vi "SignUpView.vi"(1 "Exit Button":bool) -> (0 "error out":errorcluster caption="에러 출력")   [LabVIEW 2019]
uses:
  <vilib>/Utility/miscctls.llb/LVPointTypeDef.ctl
  03_Home/controller/pannelState.ctl
panel:
  in  "signUp":bool
  out "idChecK?":bool
  in  "정지":bool
  in  "cancelBtn":bool
  in  "signUpBtn":bool
  in  "idCheck":bool
  in  "loginIdForm":string
  in  "securityAnswerForm":string
  in  "userEmailForm":string
  in  "userPhoneForm":string
  in  "userNmForm":string
  in  "passwordCheckForm":string
  in  "passwordForm":string
  in  "securityQuestionForm":string(combo)
  in  "error in (no error)":errorcluster caption="에러 입력(에러 없음)"
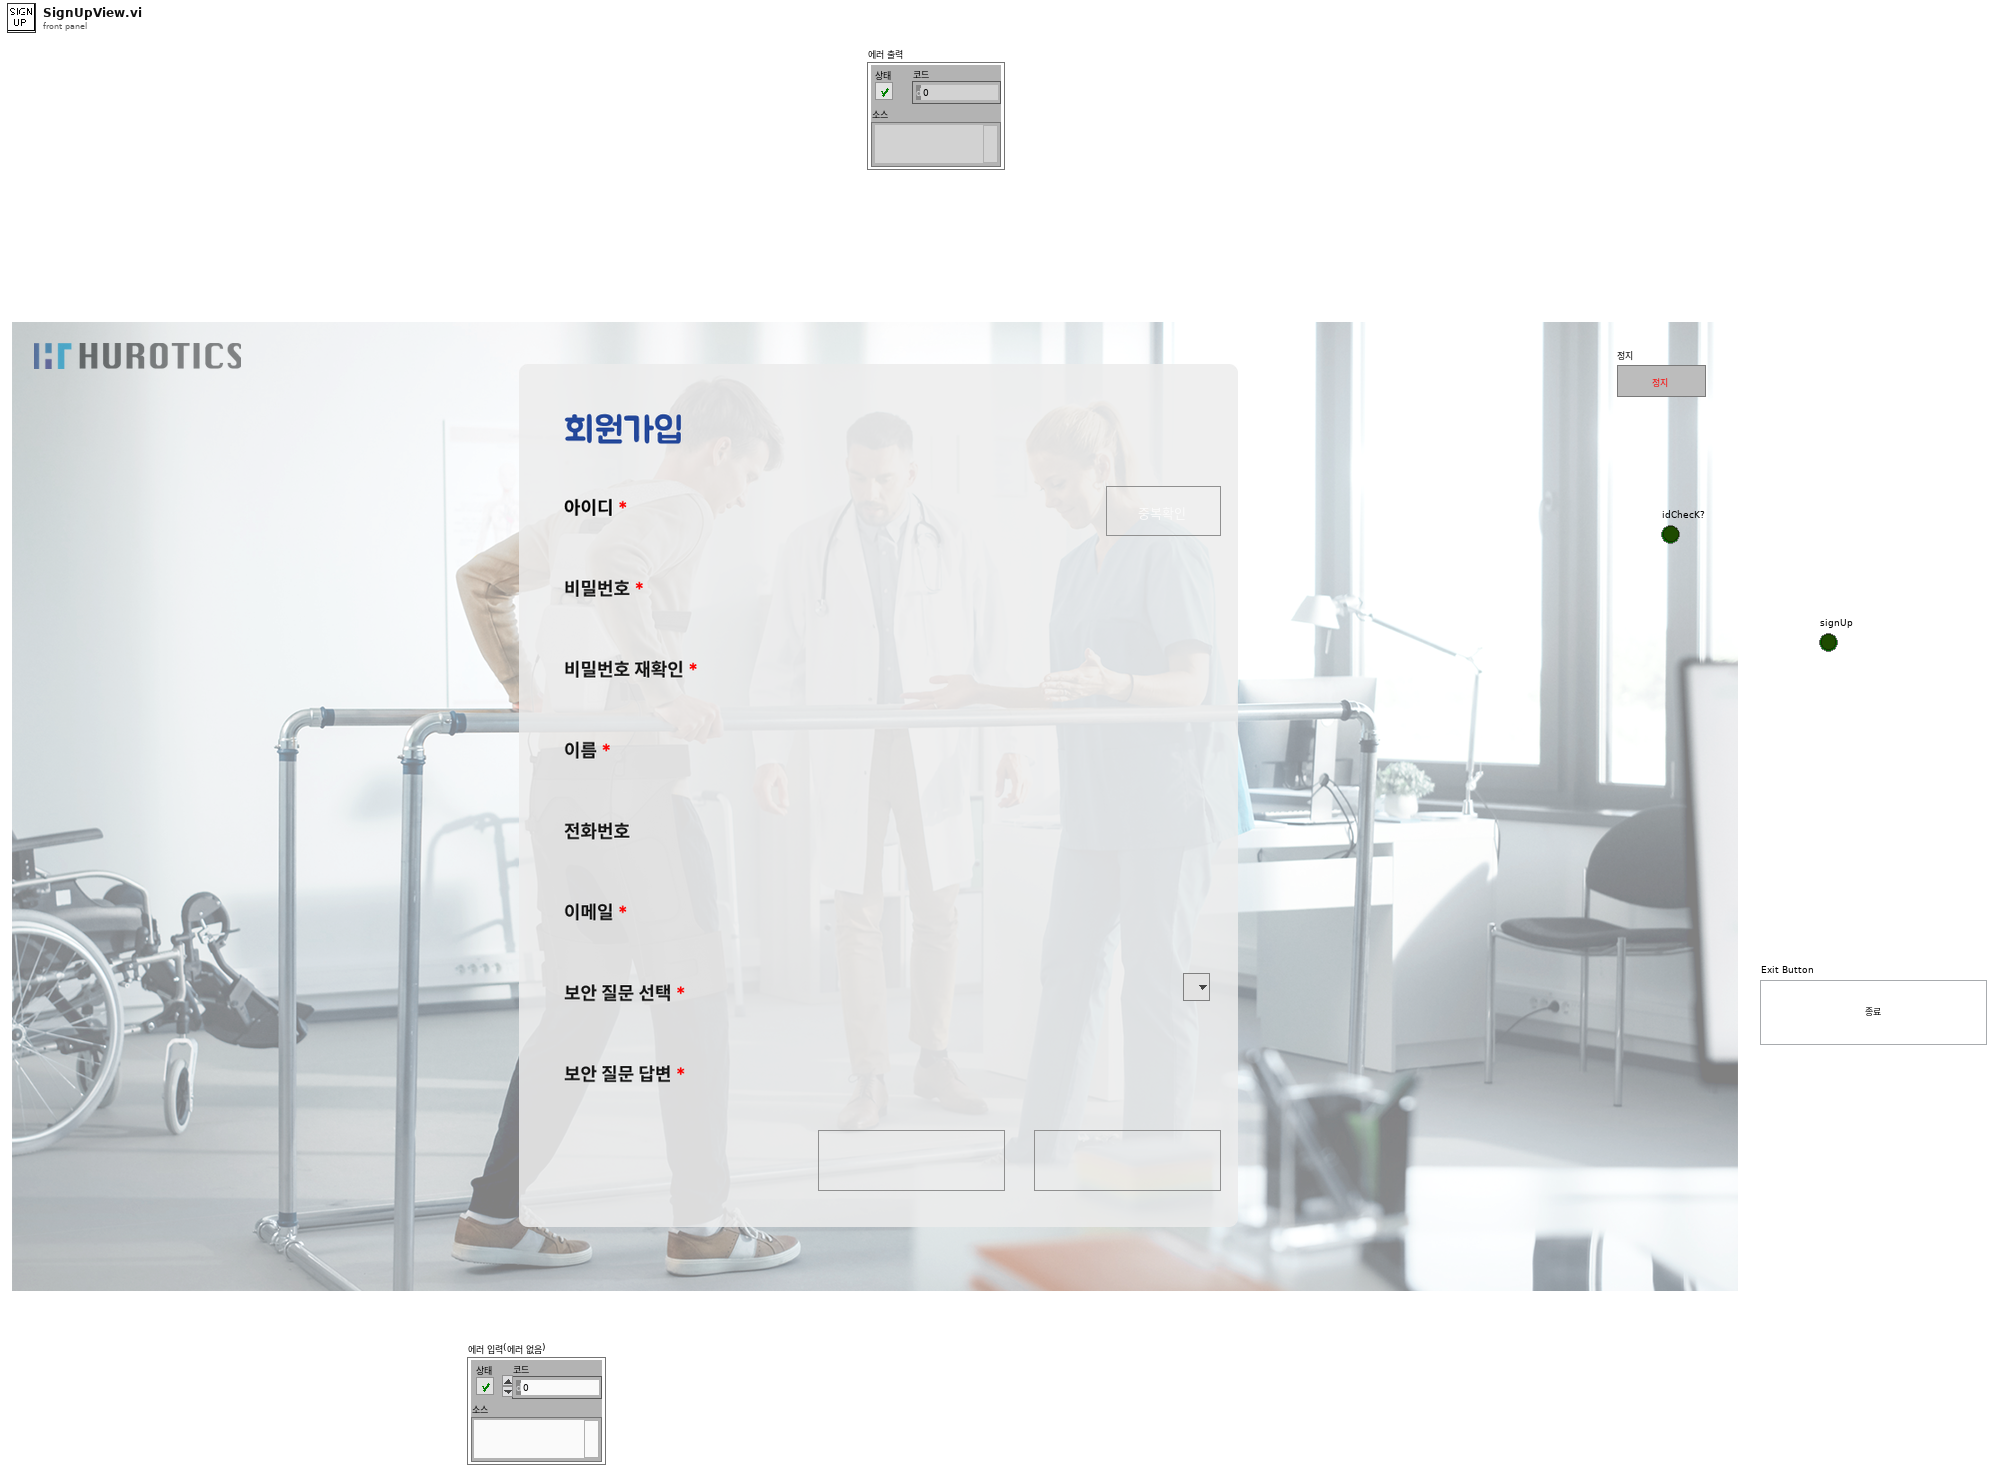
[diagram p1: front panel]
types:
  T1 = typedef "LVPointTypeDef.ctl" = cluster{"Horizontal":i16, "Vertical":i16}
  T2 = typedef "pannelState.ctl" = enum16{"Init", "LogIn", "SignUpView", "Home", "Management_patientList", "Management_patientTrashtList", "Management_patientCreate", "Management_patientUpdate", "Management_patientTraining", "Management_patientTrainingDetail", "H-MEDI PatientList", "H-MEDI HardwareCtl", "Adjust", "FineTuning", "UserList", "UserDetail", "Exit"}
  T3 = enum16{"connection", "create", "read", "update", "delete", "close"}
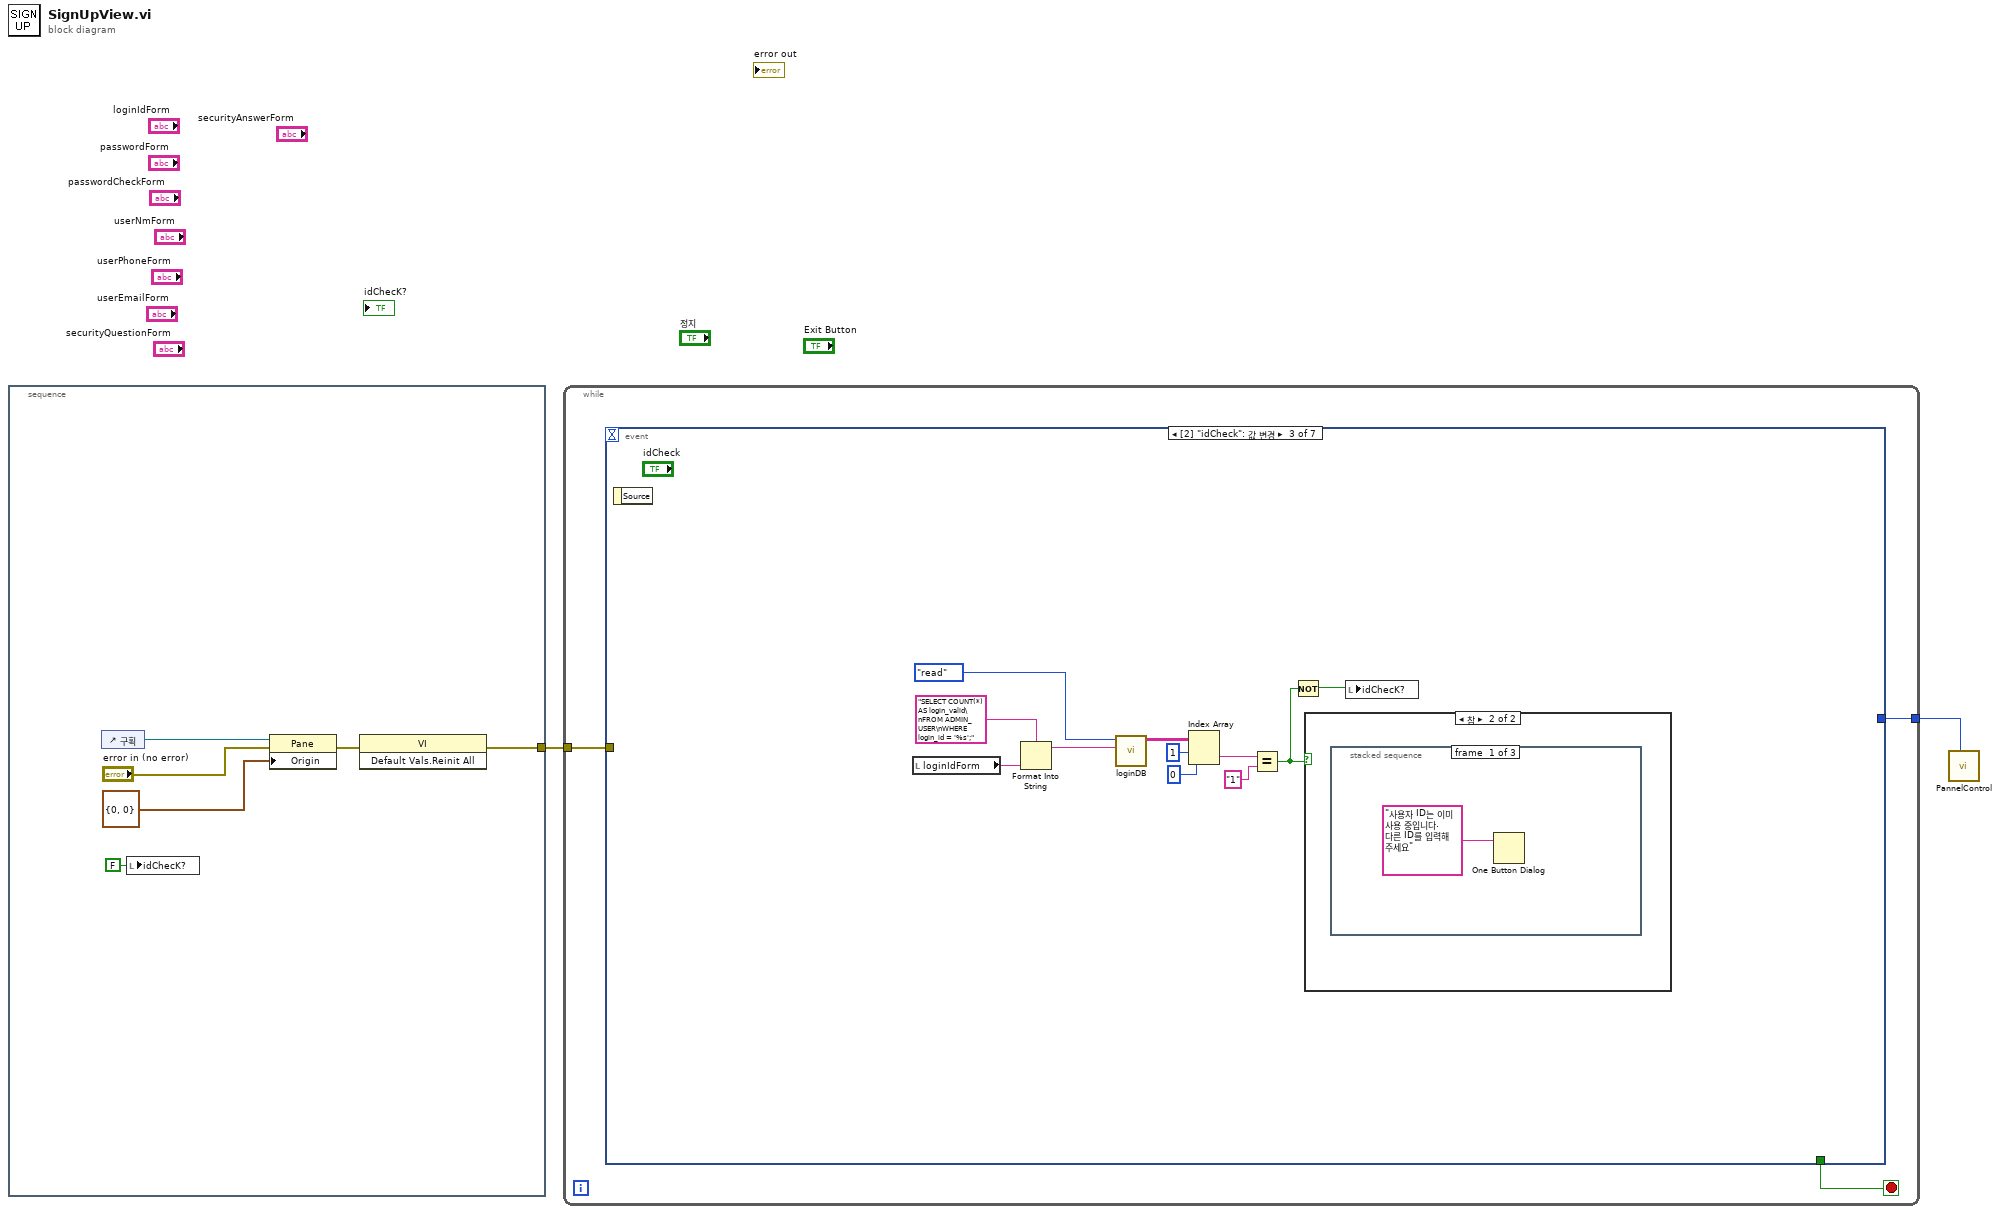
[diagram p0: block diagram]
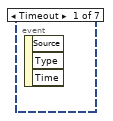
[diagram p2: hidden frame]
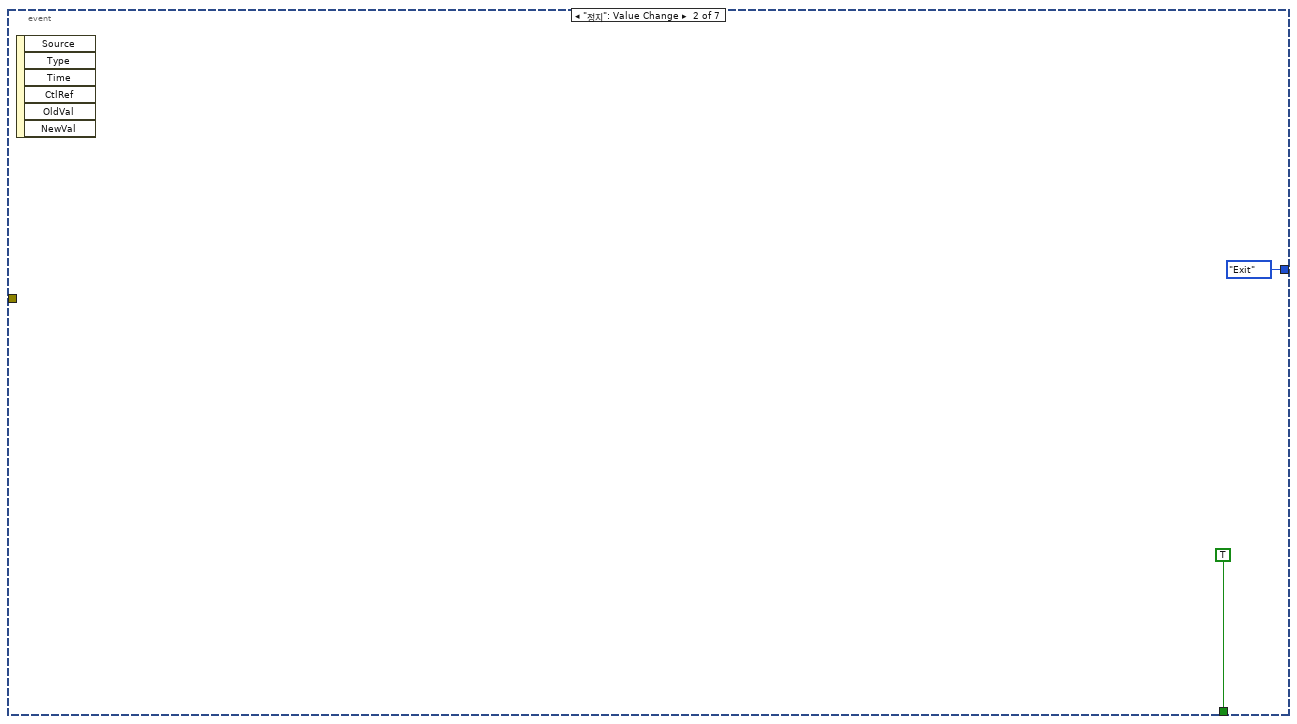
[diagram p3: hidden frame]
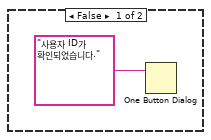
[diagram p4: hidden frame]
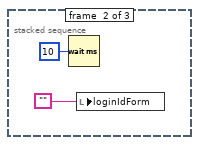
[diagram p5: hidden frame]
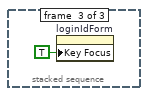
[diagram p6: hidden frame]
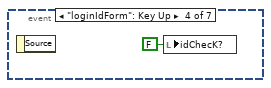
[diagram p7: hidden frame]
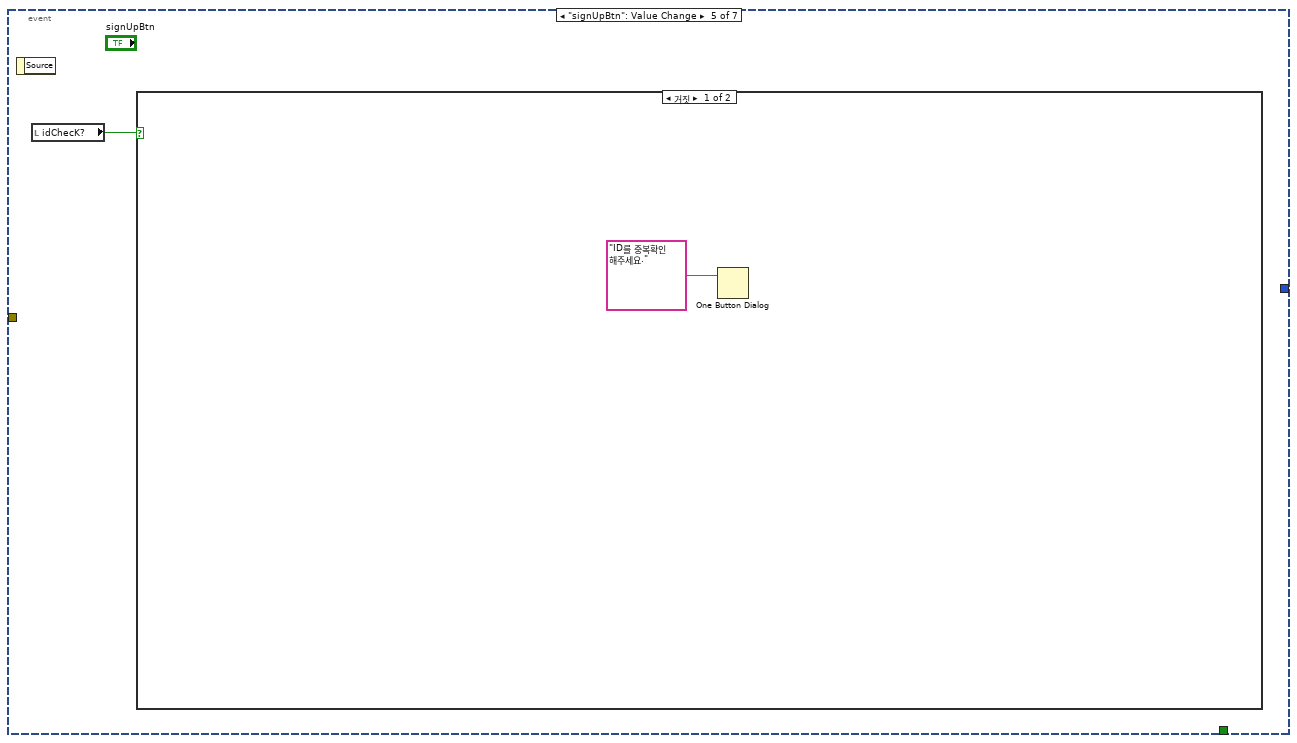
[diagram p8: hidden frame]
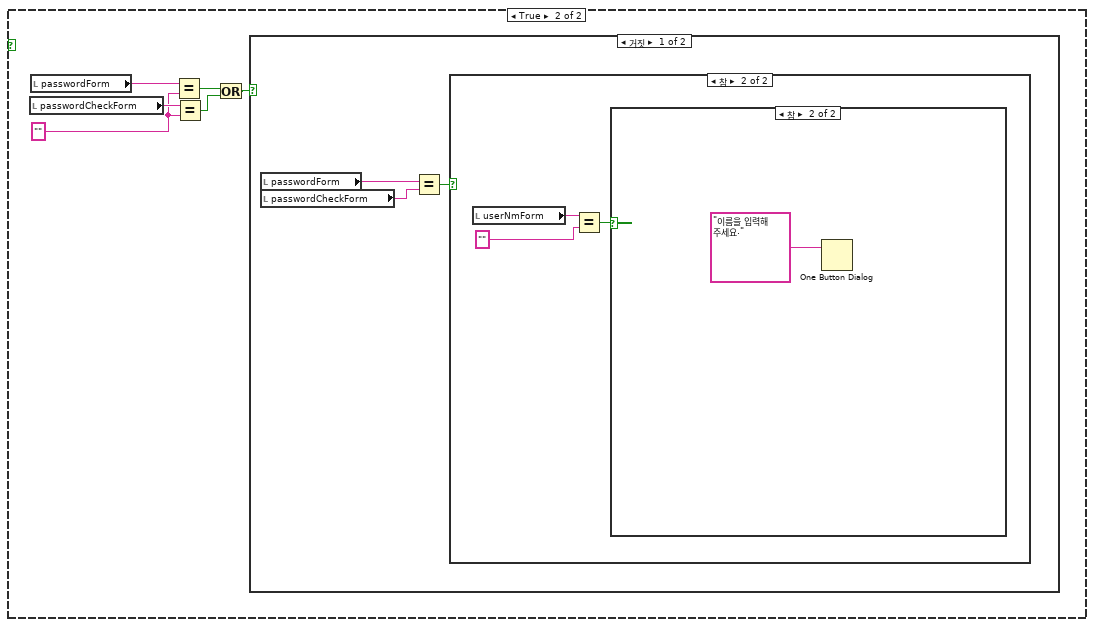
[diagram p9: hidden frame]
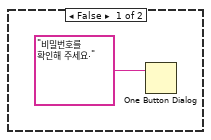
[diagram p10: hidden frame]
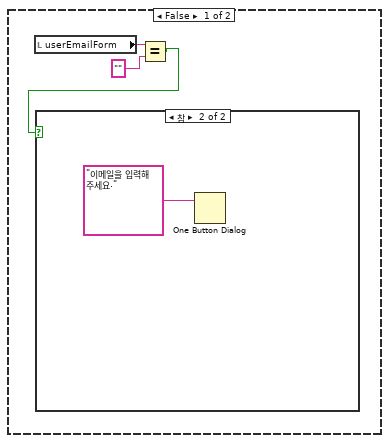
[diagram p11: hidden frame]
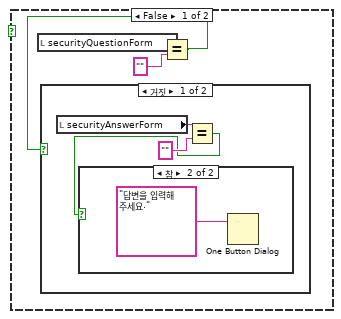
[diagram p12: hidden frame]
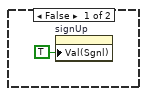
[diagram p13: hidden frame]
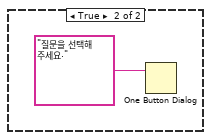
[diagram p14: hidden frame]
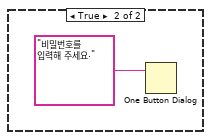
[diagram p15: hidden frame]
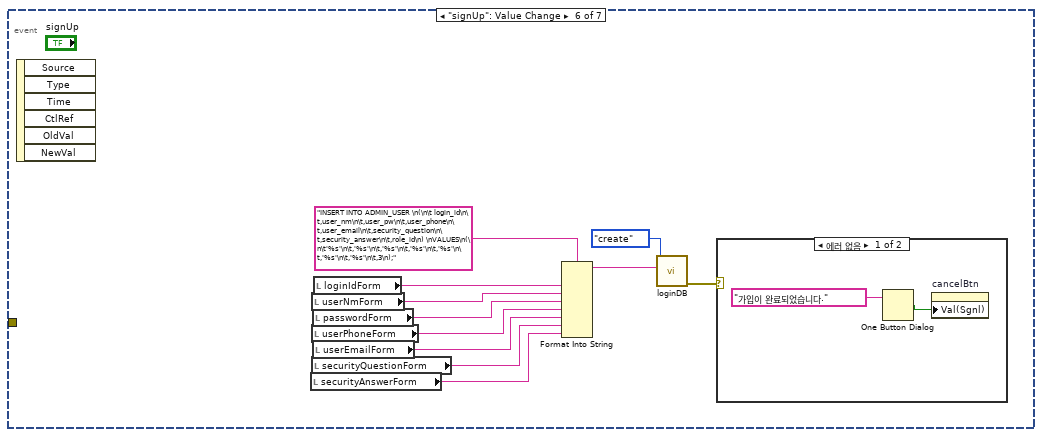
[diagram p16: hidden frame]
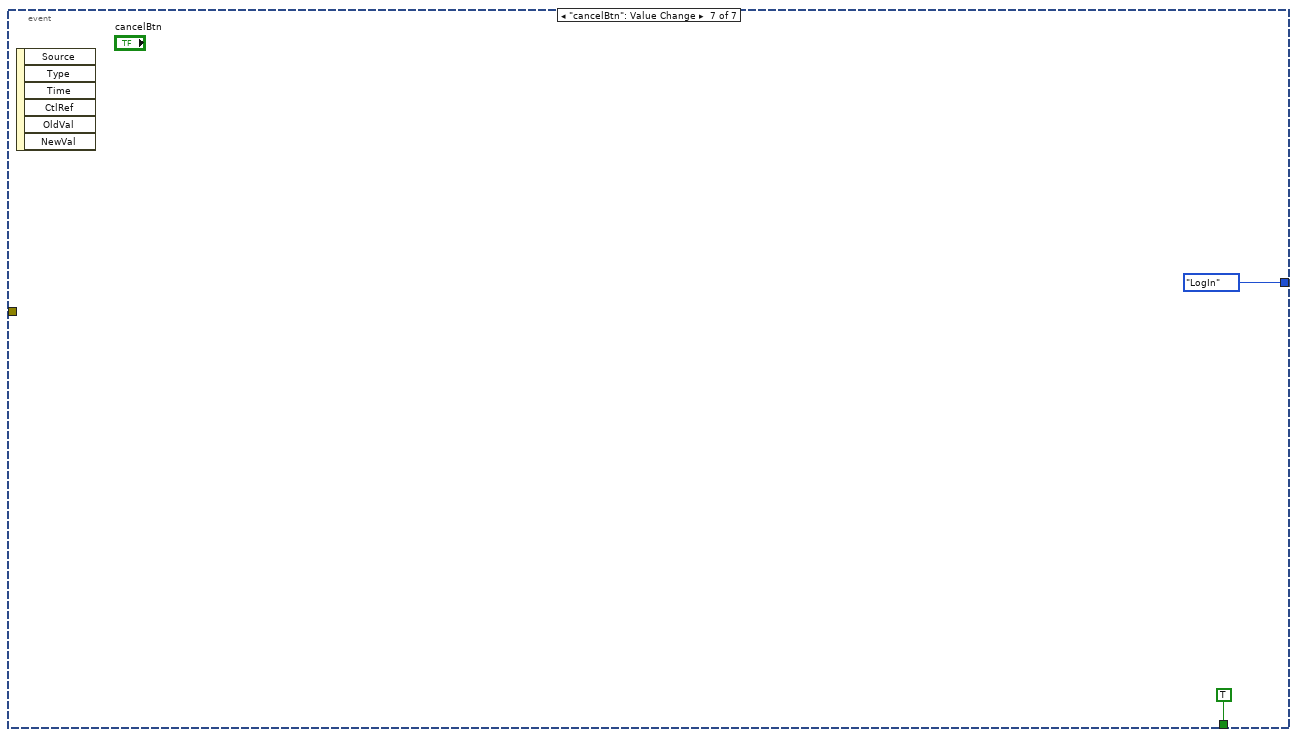
[diagram p18: hidden frame]
diagram:
  n1 = stacked-sequence {
    tunnel: [w3] -> w2
    frame #0 {
      n2 = control-ref of="구획"() -> (w7:refnum<vi>)
      n3 = local write "idChecK?"(FALSE ("idChecK?")) -> ()
      n4 = property class="Pane"(reference=w7, error in="error in (no error)", "Origin"=T1 {"Horizontal"=0, "Vertical"=0} ("원점")) -> (error out=w6:errorcluster)  [unwired: 1 out]
      n5 = invoke class="VI" method="Default Vals.Reinit All"(error in=w6) -> (error out=w3:errorcluster)  [unwired: 2 in, 2 out]
    }
  }
  n6 = while {
    tunnel: w2 -> [w10]
    tunnel: [w9] -> w1
    stop <- w11 stop-if-true
    n7 = event shown="[2] \"idCheck\": 값 변경" {
      selector: _ -> [_ _ _ _ _ _ _]
      dyn-events: _ -> [_ _ _ _ _ _ _]
      timeout: _ -> [_ _ _ _ _ _ _]
      tunnel: [_ TRUE _ _ _ _ TRUE] -> w11
      tunnel: w10 -> [_ _ _ _ _ _ _]
      tunnel: [_ pannelState."Exit" ("State") _ _ _ _ pannelState."LogIn" ("State")] -> w9
      event Timeout {
        n8 = event-data() -> ()  [unwired: 1 in, 3 out]
      }
      event "정지": Value Change {
        n9 = event-data() -> ()  [unwired: 1 in, 6 out]
      }
      event "idCheck": Value Change {
        n10 = event-data() -> ()  [unwired: 1 in, 1 out]
        n11 = local read "loginIdForm"() -> (w16:string)
        n12 = Format Into String(format string="SELECT COUNT(*) AS login_valid\nFROM ADMIN_USER\nWHERE login_id = '%s';", w16) -> (resulting string=w19:string)  [unwired: 2 in, 1 out]
        n13 = call "loginDB.vi"("Query"=w19, "State"=T3."read") -> ("Result Set"=w18:string[][])  [unwired: 7 in, 1 out]
        n14 = Index Array(array=w18, index (row)=1 ("인덱스 (행)"), index (col)=0 ("비활성화된 인덱스 (열)")) -> (element=w21:string)
        n15 = Equal?(x=w21, y="1") -> (x = y?=w15:bool)
        n16 = Not(x=w15) -> (.not. x?=w14:bool)
        n17 = case shown="참" w15 {
          frame False {
            n18 = One Button Dialog(message="사용자 ID가 확인되었습니다." ("메시지")) -> ()  [unwired: 1 in, 1 out]
          }
          frame True {
            n19 = stacked-sequence {
              frame #0 {
                n20 = One Button Dialog(message="사용자 ID는 이미 사용 중입니다. 다른 ID를 입력해 주세요" ("메시지")) -> ()  [unwired: 1 in, 1 out]
              }
              frame #1 {
                n21 = Wait (ms)(milliseconds to wait=u32 10 ("대기 시간 (ms)")) -> ()  [unwired: 1 out]
                n22 = local write "loginIdForm"("") -> ()
              }
              frame #2 {
                n23 = property on="loginIdForm" class="Str"("Key Focus"=TRUE ("키 포커스")) -> ()  [unwired: 2 in, 2 out]
              }
            }
          }
        }
        n24 = local write "idChecK?"(w14) -> ()
      }
      event "loginIdForm": Key Up {
        n25 = event-data() -> ()  [unwired: 1 in, 1 out]
        n26 = local write "idChecK?"(FALSE ("idChecK?")) -> ()
      }
      event "signUpBtn": Value Change {
        n27 = event-data() -> ()  [unwired: 1 in, 1 out]
        n28 = local read "idChecK?"() -> (w31:bool)
        n29 = case shown="거짓" w31 {
          frame False {
            n30 = One Button Dialog(message="ID를 중복확인 해주세요." ("메시지")) -> ()  [unwired: 1 in, 1 out]
          }
          frame True {
            w33 = ""
            n31 = local read "passwordCheckForm"() -> (w37:string)
            n32 = local read "passwordForm"() -> (w38:string)
            n33 = Equal?(x=w38, y=w33) -> (x = y?=w36:bool)
            n34 = Equal?(x=w37, y=w33) -> (x = y?=w35:bool)
            n35 = Or(x=w36, y=w35) -> (x .or. y?=w34:bool)
            n36 = case shown="거짓" w34 {
              frame False {
                n37 = local read "passwordForm"() -> (w41:string)
                n38 = local read "passwordCheckForm"() -> (w40:string)
                n39 = Equal?(x=w41, y=w40) -> (x = y?=w39:bool)
                n40 = case shown="참" w39 {
                  frame False {
                    n41 = One Button Dialog(message="비밀번호를 확인해 주세요." ("메시지")) -> ()  [unwired: 1 in, 1 out]
                  }
                  frame True {
                    n42 = local read "userNmForm"() -> (w45:string)
                    n43 = Equal?(x=w45, y="") -> (x = y?=w43:bool)
                    n44 = case shown="참" w43 {
                      frame False {
                        n45 = local read "userEmailForm"() -> (w47:string)
                        n46 = Equal?(x=w47, y="") -> (x = y?=w46:bool)
                        n47 = case shown="참" w46 {
                          frame False {
                            n48 = local read "securityQuestionForm"() -> (w51:string)
                            n49 = Equal?(x=w51, y="") -> (x = y?=w49:bool)
                            n50 = case shown="거짓" w49 {
                              frame False {
                                n51 = local read "securityAnswerForm"() -> (w53:string)
                                n52 = Equal?(x=w53, y="") -> (x = y?=w52:bool)
                                n53 = case shown="참" w52 {
                                frame False {
                                n54 = property on="signUp" class="Bool (엄격한)"("Val(Sgnl)"=TRUE ("값(신호)")) -> ()  [unwired: 2 in, 2 out]
                                }
                                frame True {
                                n55 = One Button Dialog(message="답변을 입력해 주세요." ("메시지")) -> ()  [unwired: 1 in, 1 out]
                                }
                                }
                              }
                              frame True {
                                n56 = One Button Dialog(message="질문을 선택해 주세요." ("메시지")) -> ()  [unwired: 1 in, 1 out]
                              }
                            }
                          }
                          frame True {
                            n57 = One Button Dialog(message="이메일을 입력해 주세요." ("메시지")) -> ()  [unwired: 1 in, 1 out]
                          }
                        }
                      }
                      frame True {
                        n58 = One Button Dialog(message="이름을 입력해 주세요." ("메시지")) -> ()  [unwired: 1 in, 1 out]
                      }
                    }
                  }
                }
              }
              frame True {
                n59 = One Button Dialog(message="비밀번호를 입력해 주세요." ("메시지")) -> ()  [unwired: 1 in, 1 out]
              }
            }
          }
        }
      }
      event "signUp": Value Change {
        n60 = event-data() -> ()  [unwired: 1 in, 6 out]
        n61 = local read "securityAnswerForm"() -> (w71:string)
        n62 = local read "userNmForm"() -> (w66:string)
        n63 = local read "userPhoneForm"() -> (w68:string)
        n64 = local read "securityQuestionForm"() -> (w70:string)
        n65 = local read "passwordForm"() -> (w67:string)
        n66 = local read "userEmailForm"() -> (w69:string)
        n67 = local read "loginIdForm"() -> (w64:string)
        n68 = Format Into String(format string="INSERT INTO ADMIN_USER \n(\n\t login_id\n\t,user_nm\n\t,user_pw\n\t,user_phone\n\t,user_email\n\t,security_question\n\t,security_answer\n\t,role_id\n) \nVALUES\n(\n\t'%s'\n\t,'%s'\n\t,'%s'\n\t,'%s'\n\t,'%s'\n\t,'%s'\n\t,'%s'\n\t,3\n);", w64, w66, w67, w68, w69, w70, w71) -> (resulting string=w65:string)  [unwired: 2 in, 1 out]
        n69 = call "loginDB.vi"("Query"=w65, "State"=T3."create") -> ("error out"=w61:errorcluster)  [unwired: 7 in, 1 out]
        n70 = case shown="에러 없음" w61 {
          frame No Error {
            n71 = One Button Dialog(message="가입이 완료되었습니다." ("메시지")) -> (true=w72:bool)  [unwired: 1 in]
            n72 = property on="cancelBtn" class="Bool (엄격한)"("Val(Sgnl)"=w72) -> ()  [unwired: 2 in, 2 out]
          }
          frame Error {
          }
        }
      }
      event "cancelBtn": Value Change {
        n73 = event-data() -> ()  [unwired: 1 in, 6 out]
      }
    }
  }
  n74 = call "PannelControl.vi"("State"=w1) -> ()  [unwired: 10 in, 1 out]
